vi "ScpSetRecordLength.vi"(8 "error in (no error)":errorcluster, 10 "u64RecordLength":u64, 11 "hDevice in":u32) -> (0 "error out":errorcluster, 2 "u64RecordLengthSet":u64, 3 "hDevice out":u32)   [LabVIEW 2018, in "LibTiePie.lvlib"]
uses:
  LibTiePie.lvlib
  LabViewHS4/libtiepie.dll
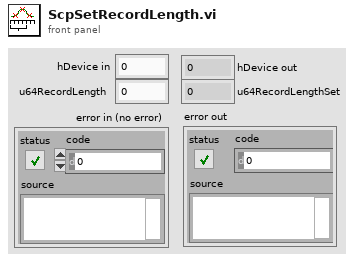
[diagram p1: front panel]
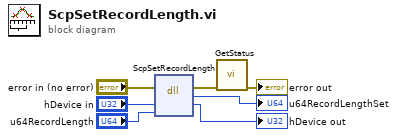
[diagram p0: block diagram]
diagram:
  n1 = dll-call lib="C:/Users/cwaha/Documents/LabViewHS4/libtiepie.dll" fn="ScpSetRecordLength"(error in="error in (no error)", "hDevice"="hDevice in", "u64RecordLength"="u64RecordLength") -> (error out=w4:errorcluster, "u64RecordLength"=→"u64RecordLengthSet":u64, "hDevice"=→"hDevice out":u32)  [unwired: 3 in, 1 out]
  n2 = call "GetStatus.vi"("error in (no error)"=w4) -> ("error out"=→"error out":errorcluster)  [unwired: 10 in]
